vi "data read make table.vi"(10 "new y-column names":string[](array[string]), 11 "Graph array":cluster{"output":dbl[], "output":dbl[]}[](array[cluster])=[{"output"=array[10000 elements], "output"=array[10000 elements]}]) -> ()   [LabVIEW 2024]
panel:
  out "spreadsheet string 2":string
  out "Array":i32[](array[numeric])
  out "spreadsheet string":string
  in  "relocate cursors":bool
  in  "analyzed data":string
  out "result":cluster{"output":dbl[], "output":dbl[]}(graph)
  in  "y-column":dbl
  in  "x-column":dbl
  out "extracted data #":i32
  in  "extracted data":string
  in  "end of input\nfor one data set":bool
  in  "menu":enum16{"subtraction"}(ring)
  in  "indice":i32[](array[numeric])
  in  "col 2":i32
  in  "col 1":i32
  in  "next data reading":bool
  out "cursor graph":cluster{"output":dbl[], "output":dbl[]}(graph)
  in  "main y-data":i32
  out "whole data set":cluster{"output":dbl[], "output":dbl[]}[](graph)
  # "For magnetothermal K analysis\nx-axis: time\ny-axis, field, Thot, Tcold, DT \nResult 1 = time, field, Thot, Tcold, DT at the cursors\nResult 2= time, field, Thot, Tcold, DT @ cursor 1, subtract 1 (cursor1-cursor1) , subtract 2 (cursor2-curso1)\n                if cursor 1 is base index."
  # "Y-column names should match"
  # "index0: base index, index i: to be compared"
  # "(1) move green cursor below onset\nyellow cursor saturation point\n(2) press stop\n(3) move the cursor set to next pts"
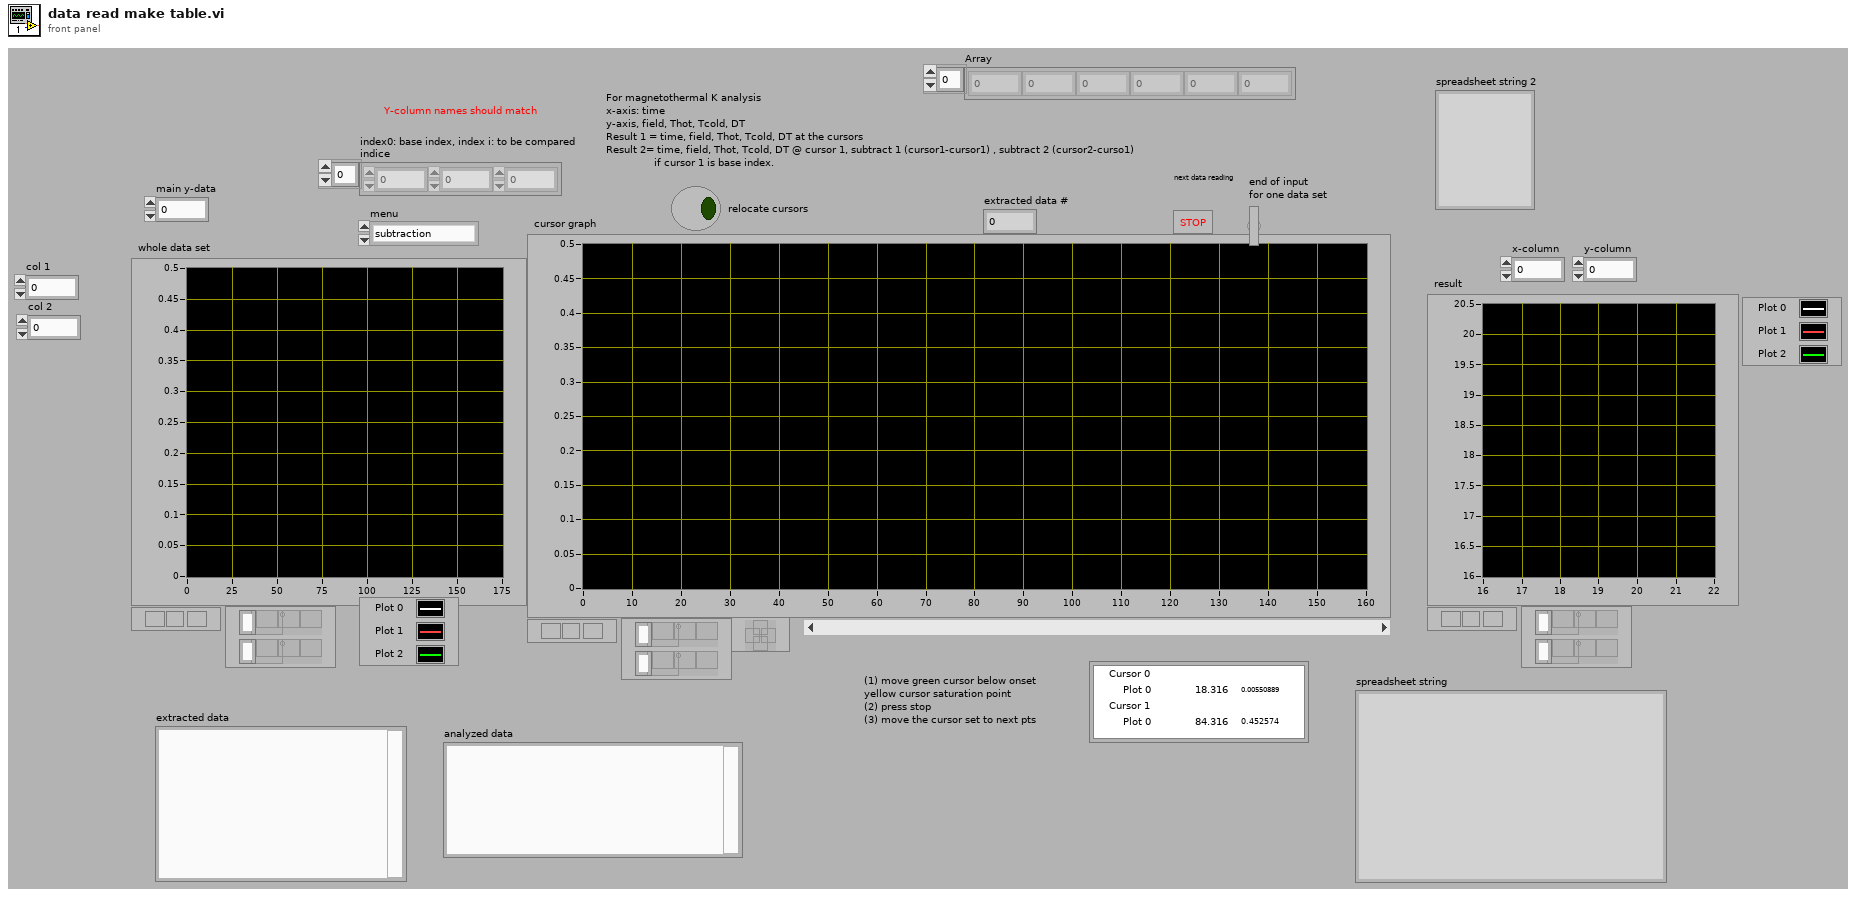
[diagram p1: front panel]
types:
  T1 = typedef "LVCursorListTypeDef.ctl" = cluster{"Name":string, "Color":u32, "Style":u8, "Point Style":u8, "Name Visible":bool, "Allow Drag":bool, "Cursor Mode":u32, "Plot":i32, "Index":i32, "Position":cluster{"X":dbl, "Y":dbl}, "X Scale":u32, "Y Scale":u32, "Watch Plots":i32[], "Watch All Plots":bool, "Plot Area":i32, "Label Offset":cluster{"X":dbl, "Y":dbl}}[]
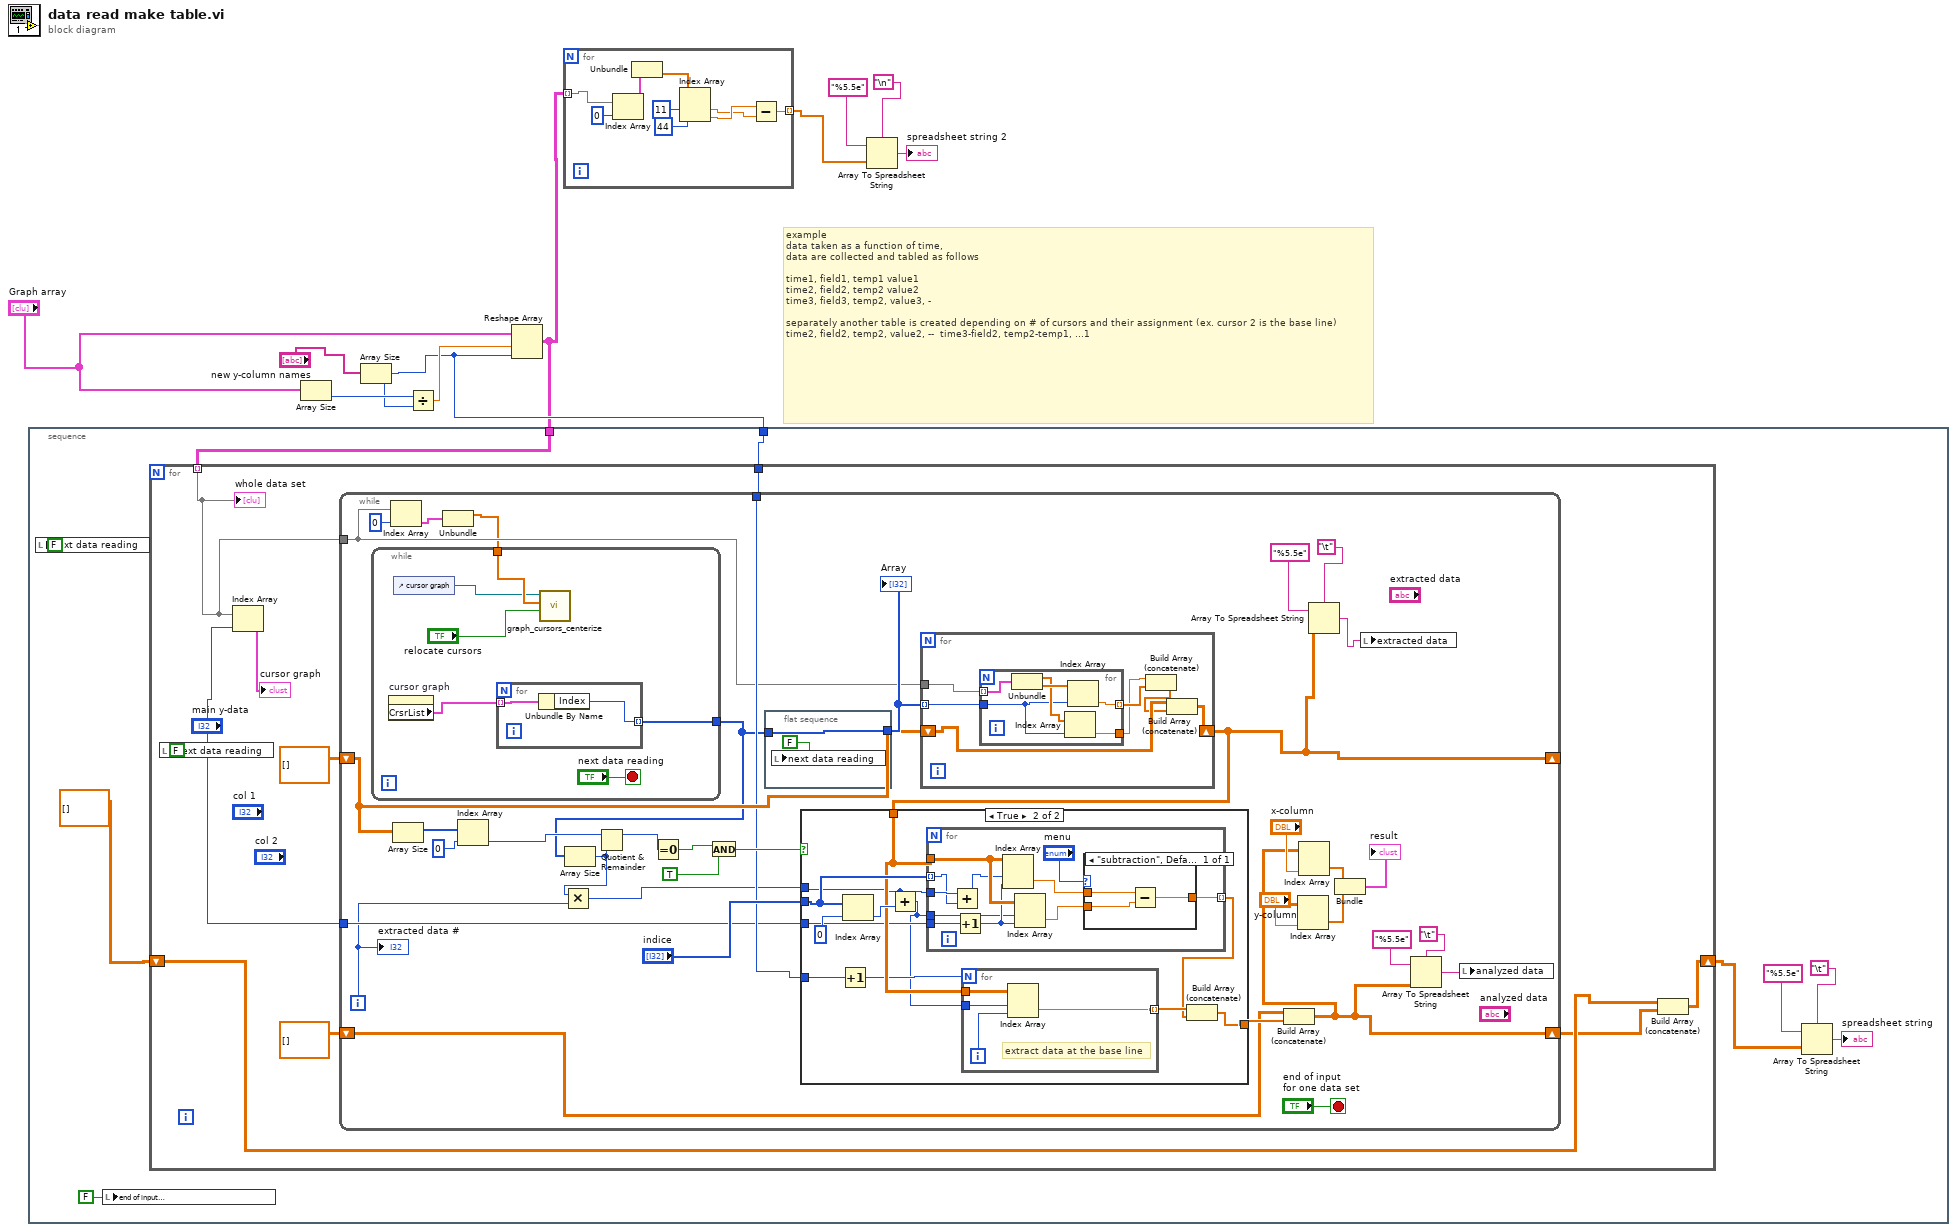
[diagram p0: block diagram]
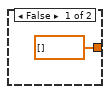
[diagram p2: hidden frame]
diagram:
  # "example\ndata taken as a function of time, \ndata are collected and tabled as follows\n\ntime1, field1, temp1 value1 \ntime2, field2, temp2 value2 \ntime3, field3, temp2, value3, -\n\nseparately another table is created depending on # of cursors and their assignment (ex. cursor 2 is the base line)\ntime2, field2, temp2, value2, --  time3-field2, temp2-temp1, ...1"
  n1 = Array Size(array="Graph array") -> (size(s)=w9:i32)
  n2 = Array Size(array="new y-column names") -> (size(s)=w7:i32)
  n3 = Divide(x=w9, y=w7) -> (x/y=w8:dbl)
  n4 = Reshape Array("Graph array", w8, w7) -> (w6:cluster{"output":dbl[], "output":dbl[]}[][])
  n5 = stacked-sequence {
    tunnel: w6 -> [w18]
    tunnel: w7 -> [w17]
    frame #0 {
      n6 = local write "next data reading"(FALSE ("stop")) -> ()
      n7 = local write "end of input\nfor one data set"(FALSE ("end of input\nfor one data set")) -> ()
      n8 = for {
        tunnel: w18 -> [w29] mode=indexing
        tunnel: w17 -> [w24]
        shift-right: [w22] -> w12
        shift-left: dbl[][] [] -> [w21]
        n9 = local write "next data reading"(FALSE ("stop")) -> ()
        n10 = Index Array(array=w29, index="main y-data") -> (element=→"cursor graph":cluster{"output":dbl[], "output":dbl[]})
        n11 = while {
          tunnel: w29 -> [w35]
          shift-right: [w39] -> _
          shift-left: dbl[][] [] -> [w54]
          shift-right: [w36] -> w20
          shift-left: dbl[][] [] -> [w57]
          tunnel: w24 -> [w47]
          tunnel: "main y-data" -> [w46]
          i -> [w44]
          stop <- "end of input\nfor one data set" stop-if-true
          n12 = Index Array(array=w35, index=0) -> (element=w33:cluster{"output":dbl[], "output":dbl[]})
          n13 = Array Size(array=w54) -> (size(s)=w65:i32[])
          n14 = Unbundle(w33) -> ("output"=w32:dbl[])  [unwired: 1 out]
          n15 = while {
            tunnel: [w115] -> w45
            tunnel: w32 -> [w114]
            stop <- "next data reading" stop-if-true
            n16 = property on="cursor graph" class="XYGraph (strict)"() -> ("CrsrList"=w116:T1)  [unwired: 2 in, 2 out]
            n17 = control-ref of="cursor graph"() -> (w113:refnum<vi>)
            n18 = for {
              tunnel: w116 -> [w119] mode=indexing
              tunnel: [w118] -> w115 mode=indexing
              n19 = Unbundle By Name(w119) -> ("Index"=w118:i32)
            }
            n20 = call "graph_cursors_centerize.vi"("centerize?"="relocate cursors", "x-axis array"=w114, "XYGraph in"=w113) -> ()  [unwired: 9 in]
          }
          n21 = Index Array(array=w65, index=0) -> (element=w63:i32)
          n22 = Array Size(array=w45) -> (size(s)=w43:i32)
          n23 = Multiply(x=w43, y=w44) -> (x*y=w42:i32)
          n24 = Quotient & Remainder(x=w63, y=w43) -> (x-y*floor(x/y)=w53:i32)  [unwired: 1 out]
          n25 = Equal To 0?(x=w53) -> (x = 0?=w61:bool)
          n26 = And(x=w61, y=TRUE) -> (x .and. y?=w62:bool)
          n27 = flat-sequence {
            tunnel: w45 -> [w67]
            tunnel: [w67] -> w56
            frame #0 {
              n28 = local write "next data reading"(FALSE ("stop")) -> ()
            }
          }
          n29 = for {
            tunnel: w35 -> [w103]
            tunnel: w56 -> [w105] mode=indexing
            shift-right: [w104] -> w39
            shift-left: w54 -> [w102]
            n30 = for {
              tunnel: w105 -> [w107]
              tunnel: [w111] -> w101 mode=indexing
              tunnel: w103 -> [w110] mode=indexing
              tunnel: [w106] -> w100
              n31 = Unbundle(w110) -> ("output"=w108:dbl[], "output"=w109:dbl[])
              n32 = Index Array(array=w108, index=w107) -> (element=w106:dbl)
              n33 = Index Array(array=w109, index=w107) -> (element=w111:dbl)
            }
            n34 = Build Array (concatenate)(w100, w101) -> (w99:dbl[])
            n35 = Build Array (concatenate)(w102, w99) -> (w104:dbl[][])
          }
          n36 = case shown="True" w62 {
            tunnel: "indice" -> [_ w79]
            tunnel: w42 -> [_ w70]
            tunnel: [dbl[] [] w75] -> w58
            tunnel: w39 -> [_ w74]
            tunnel: w47 -> [_ w73]
            tunnel: w46 -> [_ w71]
            frame False {
            }
            frame True {
              n37 = Increment(x=w73) -> (x+1=w72:i32)
              n38 = Index Array(array=w79, index=0) -> (element=w78:i32)
              n39 = Add(x=w70, y=w78) -> (x+y=w69:i32)
              n40 = for {
                tunnel: w74 -> [w95]
                tunnel: w79 -> [w89] mode=indexing
                tunnel: [w91] -> w76 mode=indexing
                tunnel: w70 -> [w90]
                tunnel: w71 -> [w87]
                tunnel: w69 -> [w85]
                n41 = Add(x=w90, y=w89) -> (x+y=w88:i32)
                n42 = Increment(x=w87) -> (x+1=w86:i32)
                n43 = Index Array(array=w95, index (row)=w88, index (col)=w86) -> (element=w93:dbl)
                n44 = Index Array(array=w95, index (row)=w85, index (col)=w86) -> (element=w92:dbl)
                n45 = case shown="\"subtraction\", Default" "menu" {
                  tunnel: w93 -> [w98]
                  tunnel: w92 -> [w97]
                  tunnel: [w96] -> w91
                  frame "subtraction", Default {
                    n46 = Subtract(x=w98, y=w97) -> (x-y=w96:dbl)
                  }
                }
              }
              n47 = for {
                N: w72 -> [_]
                tunnel: w74 -> [w84]
                tunnel: w69 -> [w83]
                tunnel: [w81] -> w77 mode=indexing
                i -> [w82]
                # "extract data at the base line"
                n48 = Index Array(array=w84, index (row)=w83, index (col)=w82) -> (element=w81:dbl)
              }
              n49 = Build Array (concatenate)(w77, w76) -> (w75:dbl[])
            }
          }
          n50 = Build Array (concatenate)(w57, w58) -> (w36:dbl[][])
          n51 = Index Array(array=w36, index (col)="y-column") -> (element=w50:dbl[])  [unwired: 1 in]
          n52 = Index Array(array=w36, index (col)="x-column") -> (element=w49:dbl[])  [unwired: 1 in]
          n53 = Array To Spreadsheet String(delimiter (Tab)="\t", array=w39, 3:"%5.5e" ("format string")) -> (spreadsheet string=w31:string)
          n54 = Bundle(w49, w50) -> (→"result":cluster{dbl[], dbl[]})  [unwired: 1 in]
          n55 = local write "extracted data"(w31) -> ()
          n56 = Array To Spreadsheet String(delimiter (Tab)="\t", array=w36, 3:"%5.5e" ("format string")) -> (spreadsheet string=w30:string)
          n57 = local write "analyzed data"(w30) -> ()
          "extracted data #" <- w44
          "Array" <- w56
        }
        n58 = Build Array (concatenate)(w21, w20) -> (w22:dbl[][])
        "whole data set" <- w29
      }
      n59 = Array To Spreadsheet String(delimiter (Tab)="\t", array=w12, 3:"%5.5e" ("format string")) -> (spreadsheet string=→"spreadsheet string":string)
    }
  }
  n60 = for {
    tunnel: w6 -> [w128] mode=indexing
    tunnel: [w120] -> w3 mode=indexing
    n61 = Index Array(array=w128, index=0) -> (element=w126:cluster{"output":dbl[], "output":dbl[]})
    n62 = Unbundle(w126) -> ("output"=w125:dbl[])  [unwired: 1 out]
    n63 = Index Array(array=w125, index #1=11 ("index"), index #2=44 ("index")) -> (element #1=w121:dbl, element #2=w122:dbl)
    n64 = Subtract(x=w122, y=w121) -> (x-y=w120:dbl)
  }
  n65 = Array To Spreadsheet String(delimiter (Tab)="\n", array=w3, 3:"%5.5e" ("format string")) -> (spreadsheet string=→"spreadsheet string 2":string)
